vi "RSZVB Set TRM Measure Input.vi"(7 "Input (At the Output)":i32(ring)=2 items=["Before the Pulse Modulator", "Before the Combiner", "At the Output"], 8 "error in (no error)":errorcluster {"code" format="%.0x"}, 9 "Path (1)":i32=1, 10 "Channel (1)":i32=1, 11 "VISA resource name":refnum<visa-resource-name>) -> (0 "error out":errorcluster {"code" format="%.0x"}, 3 "VISA resource name out":refnum<visa-resource-name>)   [LabVIEW 2011]
doc: "This VI selects the input for the a-wave (REF) receiver at paths no. 1-4.\n\nRemote-control command(s):\n[SENSe<Ch>:]TEUNit:AMONitor<Path>"
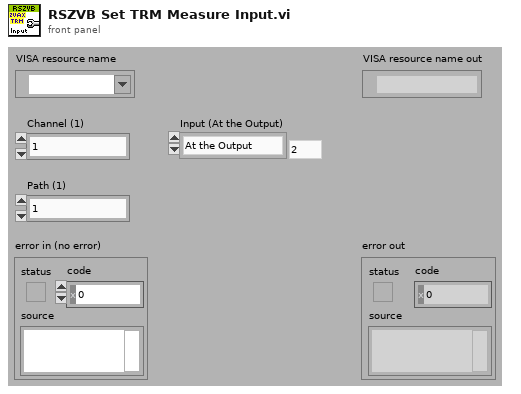
[diagram p1: front panel]
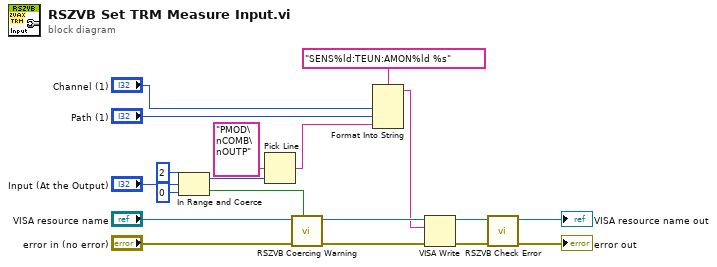
[diagram p0: block diagram]
diagram:
  n1 = In Range and Coerce(upper limit=2, x="Input (At the Output)", lower limit=0) -> (coerced(x)=w6:i32, In Range?=w10:bool)
  n2 = Pick Line(multi-line string="PMOD\nCOMB\nOUTP", line index=w6) -> (output string=w5:string)  [unwired: 1 in]
  n3 = call "RSZVB Coercing Warning.vi"("In Range?"=w10, "error in (no error)"="error in (no error)", "VISA session"="VISA resource name") -> ("error out"=w18:errorcluster, "dup VISA session"=w19:refnum<visa-resource-name>)  [unwired: 7 in]
  n4 = Format Into String(format string="SENS%ld:TEUN:AMON%ld %s", "Channel (1)", "Path (1)", w5) -> (resulting string=w1:string)  [unwired: 2 in, 1 out]
  n5 = VISA Write(VISA resource name=w19, write buffer=w1, error in (no error)=w18) -> (VISA resource name out=w16:refnum<visa-resource-name>, error out=w17:errorcluster)  [unwired: 1 out]
  n6 = call "RSZVB Check Error.vi"("error in (no error)"=w17, "VISA session"=w16) -> ("error out"=→"error out":errorcluster, "dup VISA session"=→"VISA resource name out":refnum<visa-resource-name>)  [unwired: 8 in]
